vi "boolean latch.vi"(9 "clear":bool, 11 "set":bool) -> (3 "out":bool)   [LabVIEW 2018, in "tools.lvlib"]
uses:
  tools.lvlib
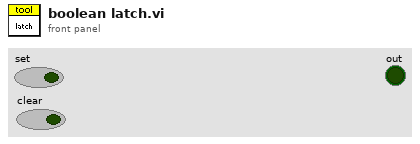
[diagram p1: front panel]
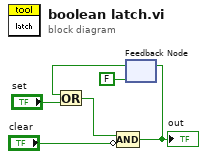
[diagram p0: block diagram]
diagram:
  n1 = feedback #1(FALSE) -> (w1:bool)
  n2 = Or(x=w1, y="set") -> (x .or. y?=w6:bool)
  n3 = Compound Arithmetic op=AND(w6, invert "clear") -> (w5:bool)
  "out" <- w5
  n4 = feedback-in #1(w5) -> ()
